vi "csmdoc_export_all_csm_VI_description_doc.vi"(11 "Path":path=path "D:/github/JKI-State-Machine-Plus/.doc/VI Description.md") -> ()   [LabVIEW 2017, in "csmdoc.lvlib"]
uses:
  csmdoc.lvlib
  Communicable State Machine.lvlib
panel:
  in  "Error in":errorcluster caption="Error in (no error)"
  out "error out":errorcluster
  out "Array":path[](array[path])
  out "concatenated string":string
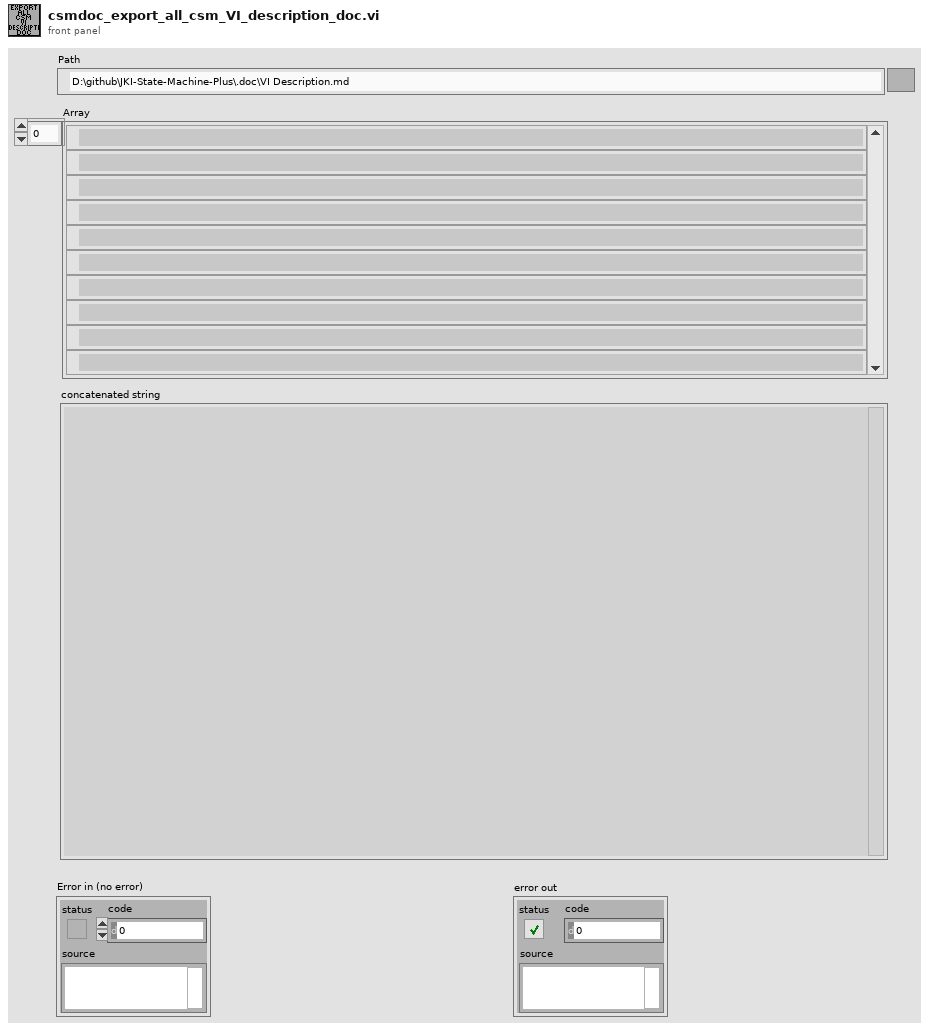
[diagram p1: front panel]
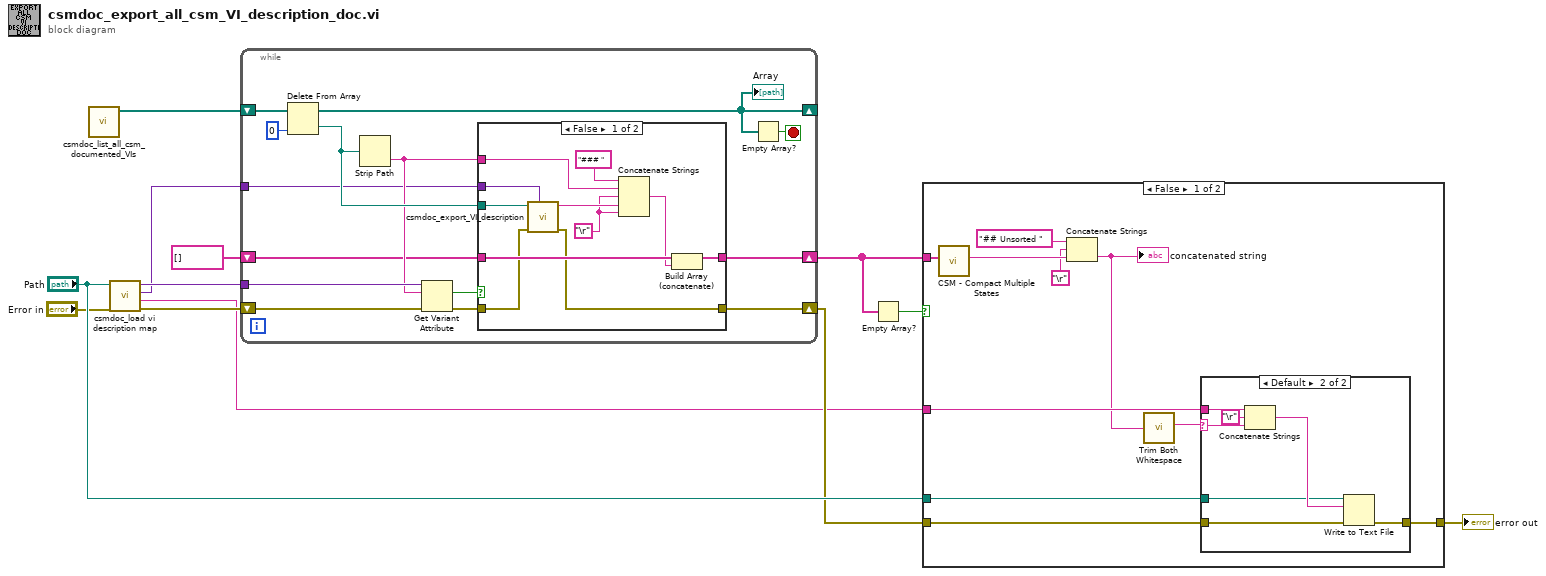
[diagram p0: block diagram]
diagram:
  n1 = call "csmdoc_list_all_csm_documented_VIs.vi"() -> ("Array"=w12:path[])  [unwired: 11 in]
  n2 = call "csmdoc_load vi description map.vi"("Error in"="Error in", "Path"="Path") -> ("Error out"=w8:errorcluster, "text"=w6:string, "variant 2"=w1:variant, "variant"=w11:variant)  [unwired: 6 in]
  n3 = while {
    shift-right: [w23] -> _
    shift-left: w12 -> [w25]
    tunnel: w11 -> [w21]
    shift-right: [w18] -> w3
    shift-left: string[] [] -> [w17]
    shift-right: [w14] -> w7
    shift-left: w8 -> [w16]
    tunnel: w1 -> [w13]
    stop <- w24 stop-if-true
    n4 = Delete From Array(array=w25, index=0) -> (deleted portion=w26:path, array with subset deleted=w23:path[])  [unwired: 1 in]
    "Array" <- w23
    n5 = Strip Path(path=w26) -> (name=w20:string)  [unwired: 1 out]
    n6 = Get Variant Attribute(Variant=w21, name=w20, error in=w16) -> (found=w19:bool, error out=w15:errorcluster)  [unwired: 1 in, 2 out]
    n7 = case shown="False" w19 {
      tunnel: w26 -> [w34 _]
      tunnel: w20 -> [w33 _]
      tunnel: [w31 w39] -> w18
      tunnel: w17 -> [w32 w39]
      tunnel: w15 -> [w29 w38]
      tunnel: [w28 w38] -> w14
      tunnel: w13 -> [w27 _]
      frame False {
        w35 = "\r"
        n8 = call "csmdoc_export_VI_description.vi"("NOTE-Map"=w27, "error in (no error)"=w29, "Path"=w34) -> ("error out"=w28:errorcluster, "concatenated string"=w37:string)  [unwired: 7 in]
        n9 = Concatenate Strings("### " ("string"), w33, w35, w37, w35) -> (w30:string)
        n10 = Build Array (concatenate)(w32, w30) -> (w31:string[])
      }
      frame True {
      }
    }
    n11 = Empty Array?(array=w23) -> (empty?=w24:bool)
  }
  n12 = Empty Array?(array=w3) -> (empty?=w2:bool)
  n13 = case shown="False" w2 {
    tunnel: "Path" -> [w45 _]
    tunnel: w7 -> [w44 w58]
    tunnel: w6 -> [w43 _]
    tunnel: [w41 w58] -> w5
    tunnel: w3 -> [w40 _]
    frame False {
      n14 = call "CSM - Compact Multiple States.vi"("Multiple States"=w40) -> ("States"=w48:string)  [unwired: 9 in]
      n15 = Concatenate Strings("## Unsorted " ("string"), "\r" ("Carriage Return Constant"), w48) -> (w42:string)
      "concatenated string" <- w42
      n16 = call "Trim Both Whitespace.vi"("string"=w42) -> ("trimmed string"=w46:string)  [unwired: 1 in]
      n17 = case shown="Default" w46 {
        selector: w46 -> [_ w56]
        tunnel: w43 -> [_ w55]
        tunnel: w45 -> [_ w53]
        tunnel: w44 -> [w50 w52]
        tunnel: [w50 w51] -> w41
        frame "" {
        }
        frame Default {
          n18 = Concatenate Strings(w55, "\r", w56) -> (w54:string)
          n19 = Write to Text File(file (use dialog)=w53, text=w54, error in=w52) -> (error out=w51:errorcluster)  [unwired: 1 in, 2 out]
        }
      }
    }
    frame True {
    }
  }
  "error out" <- w5
